vi "Set Scheduled Message Data.vi"(8 "error in (no error)":errorcluster, 10 "value":u32 format="%08x", 11 "message handle in":u64) -> (0 "error out":errorcluster, 3 "message handle out":u64)   [LabVIEW 2020, in "Ballard ARINC 429 Hardware API.lvlib"]
doc: "This VI operates on a single message. If multiple messages need to be accessed, it begins to make sense to use the batched alternative to this VI for a performance improvement, <B>Set Scheduled Message Group Data</B>. The number of messages varies by application, but a reasonable starting point is 4.\n\nSets the message data associated with <B>message handle in</B>. This VI updates the data associated with a current-value message and replaces all data with a single data item in FIFO message lists. Updating message list data for circular message lists will fail.\n\nThe exact bits that get updated in the message depend on how the message has been defined in the configuration file. If <B>labelDecimal</B> is defined, the 8 corresponding to the label will be masked off and not updated by this VI. If <B>SDI</B> is defined or not set to \"Off\", the 2 bits corresponding to the SDI field will be masked off and not updated by this VI.\n\nMessages that have never been written to from the application will be initialized with 0's by default, but the configuration file is capable of changing this via the <B>dataWipe</B> attribute or by data initialized via the <B>rawData</B> element under the associated <B>messageBuffer</B> element."
uses:
  Ballard ARINC 429 Hardware API.lvlib
  BTI429LV.dll
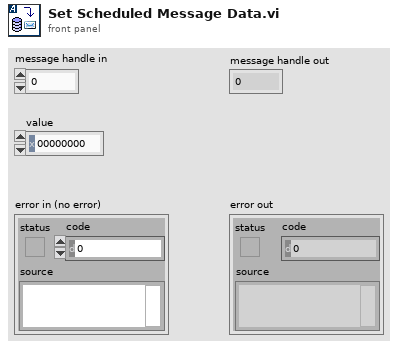
[diagram p1: front panel]
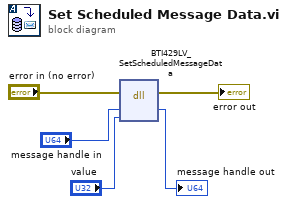
[diagram p0: block diagram]
diagram:
  n1 = dll-call lib="BTI429LV.*" fn="BTI429LV_SetScheduledMessageData"(error in="error in (no error)", "msghandle"="message handle in", "value"="value") -> (error out=→"error out":errorcluster, "msghandle"=→"message handle out":u64)  [unwired: 4 in, 1 out]
